vi "Update Legend.vi"(8 "error in (no error)":errorcluster, 10 "Legend":T1={"Enable"=FALSE, "Title"="", "TitleSeparator"=enum."None", "Over Plot?"=FALSE, "Docking"=enum."Top", "Border"={"color"={"Color"=0, "alpha"=76}, "DashStyle"=enum."NotSet", "Width"=2}, "Background"={"Color"={"Color"=0, "alpha"=76}, "HatchStyle"=76, "GradientStyle"=0}, "font"={"Name"="Arial", "Size"=16.0, "style"=0, "Color"={"Color"=0, "alpha"=76}}} {"font"."Color"."alpha" scale=0.0..255.0; "font"."style" items=["Regular"=0, "Bold"=1, "Italic"=2, "Underline"=4, "Strikeout"=8]; "font"."Size" min=4.0 max=100.0; "Background"."GradientStyle" items=["None", "LeftRight", "TopBottom", "Center", "DiagonalLeft", "DiagonalRight", "HorizontalCenter", "VerticalCenter"]; "Background"."HatchStyle" items=["None", "BackwardDiagonal", "Cross", "DarkDownwardDiagonal", "DarkHorizontal", "DarkUpwardDiagonal", "DarkVertical", "DashedDownwardDiagonal", "DashedHorizontal", "DashedUpwardDiagonal", "DashedVertical", "DiagonalBrick", "DiagonalCross", "Divot", "DottedDiamond", "DottedGrid", "ForwardDiagonal", "Horizontal", "HorizontalBrick", "LargeCheckerBoard", "LargeConfetti", "LargeGrid", "LightDownwardDiagonal", "LightHorizontal", "LightUpwardDiagonal", "LightVertical", "NarrowHorizontal", "NarrowVertical", "OutlinedDiamond", "Percent05", "Percent10", "Percent20", "Percent25", "Percent30", "Percent40", "Percent50", "Percent60", "Percent70", "Percent75", "Percent80", "Percent90", "Plaid", "Shingle", "SmallCheckerBoard", "SmallConfetti", "SmallGrid", "SolidDiamond", "Sphere", "Trellis", "Vertical", "Wave", "Weave", "WideDownwardDiagonal", "WideUpwardDiagonal", "ZigZag"]; "Background"."Color"."alpha" scale=0.0..255.0; "Border"."color"."alpha" scale=0.0..255.0}, 11 ".NET MSChart Legend In":refnum<k24>) -> (0 "error out":errorcluster, 3 ".NET MSChart Legend":refnum<k24>)   [LabVIEW 2014, in "XMSChart.xctl"]
uses:
  XMSChart.xctl
  System.Windows.Forms.DataVisualization
  Controls/Legend.ctl
  Controls/Border.ctl
  Controls/Color.ctl
  Controls/Background.ctl
  Controls/Font.ctl
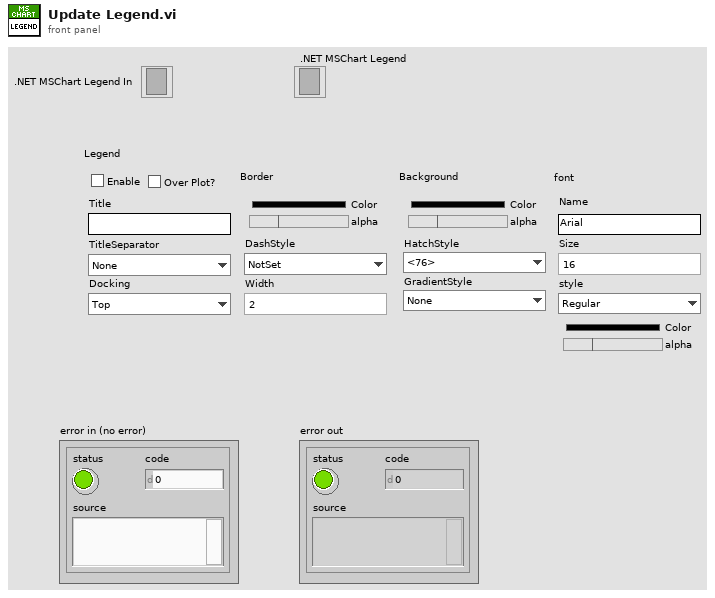
[diagram p1: front panel]
types:
  T1 = typedef "XMSChart.xctl/Legend.ctl" = cluster{"Enable":bool, "Title":string, "TitleSeparator":enum16{"None", "Line", "ThickLine", "DoubleLine", "DashLine", "DotLine", "GradientLine", "ThickGradientLine"}, "Over Plot?":bool, "Docking":enum16{"Top", "Right", "Bottom", "Left", "None"}, "Border":T2, "Background":T4, "font":T5}
  T2 = typedef "XMSChart.xctl/Border.ctl" = cluster{"color":T3, "DashStyle":enum16{"NotSet", "Dash", "DashDot", "DashDotDot", "Dot", "Solid"}, "Width":i32}
  T3 = typedef "XMSChart.xctl/Color.ctl" = cluster{"Color":u32, "alpha":u8}
  T4 = typedef "XMSChart.xctl/Background.ctl" = cluster{"Color":T3, "HatchStyle":i32, "GradientStyle":i32}
  T5 = typedef "XMSChart.xctl/Font.ctl" = cluster{"Name":string, "Size":dbl, "style":i32, "Color":T3}
  T6 = enum16{"None", "Line", "ThickLine", "DoubleLine", "DashLine", "DotLine", "GradientLine", "ThickGradientLine"}
  T7 = enum16{"NotSet", "Dash", "DashDot", "DashDotDot", "Dot", "Solid"}
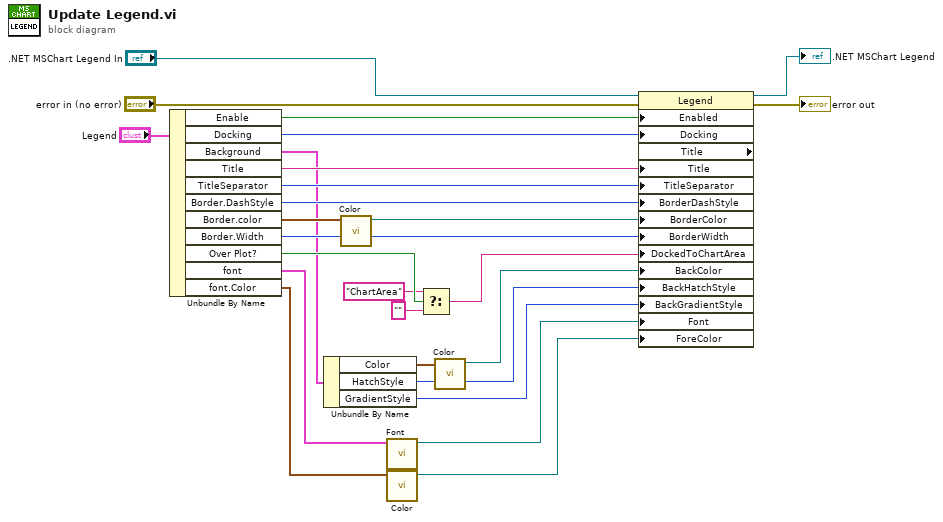
[diagram p0: block diagram]
diagram:
  n1 = Unbundle By Name("Legend") -> ("Enable"=w5:bool, "Docking"=w12:enum16{"Top", "Right", "Bottom", "Left", "None"}, "Background"=w10:T4, "Title"=w23:string, "TitleSeparator"=w22:T6, "Border.DashStyle"=w20:T7, "Border.color"=w17:T3, "Border.Width"=w19:i32, "Over Plot?"=w16:bool, "font"=w4:T5, "font.Color"=w2:T3)
  n2 = Unbundle By Name(w10) -> ("Color"=w9:T3, "HatchStyle"=w7:i32, "GradientStyle"=w6:i32)
  n3 = call "Color.vi"("BGK Color"=w17) -> (".NET Refnum out"=w18:refnum<k24>)  [unwired: 10 in]
  n4 = call "Font.vi"("font"=w4) -> (".NET MSChart Font"=w3:refnum<k24>)  [unwired: 10 in]
  n5 = call "Color.vi"("BGK Color"=w2) -> (".NET Refnum out"=w1:refnum<k24>)  [unwired: 10 in]
  n6 = Select(t="ChartArea" ("DockedToChartArea"), s=w16, f="") -> (s? t:f=w13:string)
  n7 = call "Color.vi"("BGK Color"=w9) -> (".NET Refnum out"=w8:refnum<k24>)  [unwired: 10 in]
  n8 = property on="Property Node" class="Legend" props=["Enabled", "Docking", "Title", "Title", "TitleSeparator", "BorderDashStyle", "BorderColor", "BorderWidth", "DockedToChartArea", "BackColor", "BackHatchStyle", "BackGradientStyle", "Font", "ForeColor"](reference=".NET MSChart Legend In", error in="error in (no error)", "Enabled"=w5, "Docking"=w12, "Title"=w23, "TitleSeparator"=w22, "BorderDashStyle"=w20, "BorderColor"=w18, "BorderWidth"=w19, "DockedToChartArea"=w13, "BackColor"=w8, "BackHatchStyle"=w7, "BackGradientStyle"=w6, "Font"=w3, "ForeColor"=w1) -> (reference out=→".NET MSChart Legend":refnum<k24>, error out=→"error out":errorcluster)  [unwired: 1 out]
